vi "Shallow Copy and Deep Copy.vi"() -> ()   [LabVIEW 2020, in "NI_VIAnCFGDataStructure.lvlib" / "Tree.lvclass"]
uses:
  <vilib>/addons/analyzer/VIAnCFGDataStructure/Tree Manager/Tree.lvclass
  <vilib>/addons/analyzer/VIAnCFGDataStructure/Data Types/Int/Int.lvclass/Int.ctl
  <vilib>/addons/analyzer/VIAnCFGDataStructure/Data Types/Path/Path.lvclass/Path.ctl
  <vilib>/addons/analyzer/VIAnCFGDataStructure/Data Types/String/String.lvclass/String.ctl
  <vilib>/addons/analyzer/VIAnCFGDataStructure/Data Types/Path/To Path Tree Data.vi
  <vilib>/addons/analyzer/VIAnCFGDataStructure/Data Types/String/To String Tree Data.vi
  <vilib>/addons/analyzer/VIAnCFGDataStructure/Data Types/Int/To Integer Tree Data.vi
  <vilib>/addons/analyzer/VIAnCFGDataStructure/Data Types/Int/Int.lvclass
  e:/builds/penguin/labview/branches/2020/dev/dist/vi.lib/addons/analyzer/VIAnCFGDataStructure/Tree Data/Tree Data.lvclass
  <vilib>/addons/analyzer/VIAnCFGDataStructure/Data Types/String/String.lvclass
  <vilib>/addons/analyzer/VIAnCFGDataStructure/Data Types/Path/Path.lvclass
  <vilib>/addons/analyzer/VIAnCFGDataStructure/Tree Manager/API/Set Attribute Tree Data.vi
  e:/builds/penguin/labview/branches/2020/dev/dist/vi.lib/addons/analyzer/VIAnCFGDataStructure/Data Types/Int/Int.lvclass
  e:/builds/penguin/labview/branches/2020/dev/dist/vi.lib/addons/analyzer/VIAnCFGDataStructure/Data Types/String/String.lvclass
  e:/builds/penguin/labview/branches/2020/dev/dist/vi.lib/addons/analyzer/VIAnCFGDataStructure/Data Types/Path/Path.lvclass
panel:
  in  "Show IDs (True)":bool
  in  "After Deep Copy":string(tree)
  in  "After Shallow Copy":string(tree)
  in  "Before Copy":string(tree)
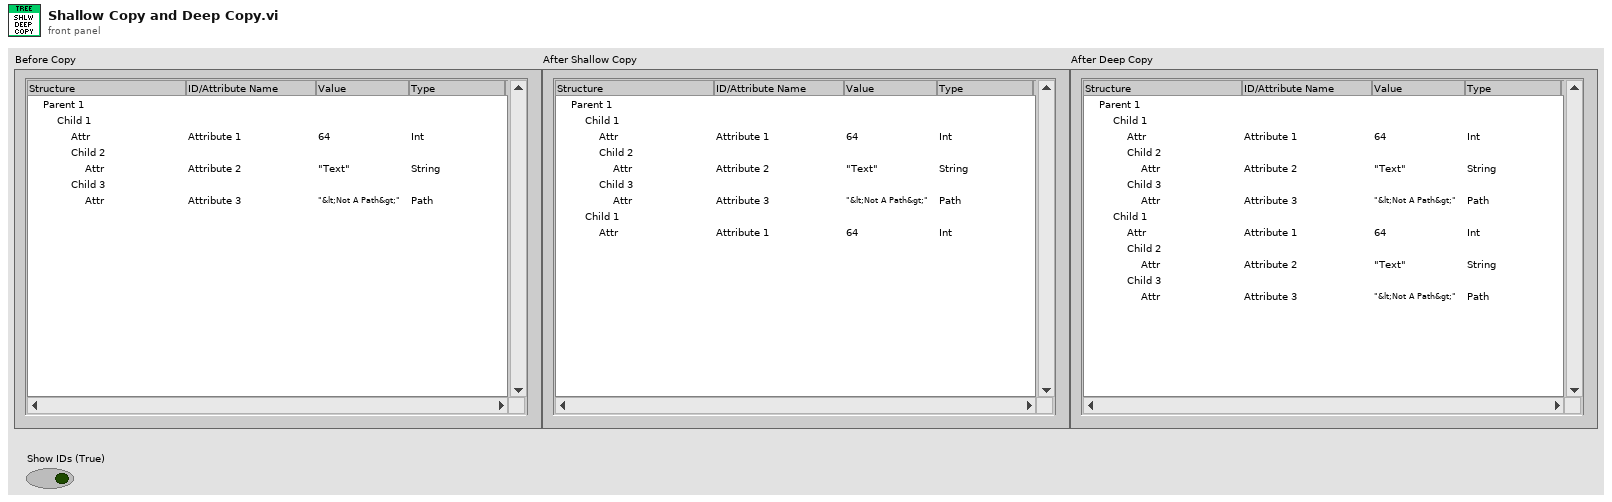
[diagram p1: front panel]
types:
  T1 = typedef "NI_VIAnCFGDataStructure.lvlib/Tree.lvclass/Session Handle.ctl" = refnum<data-value>
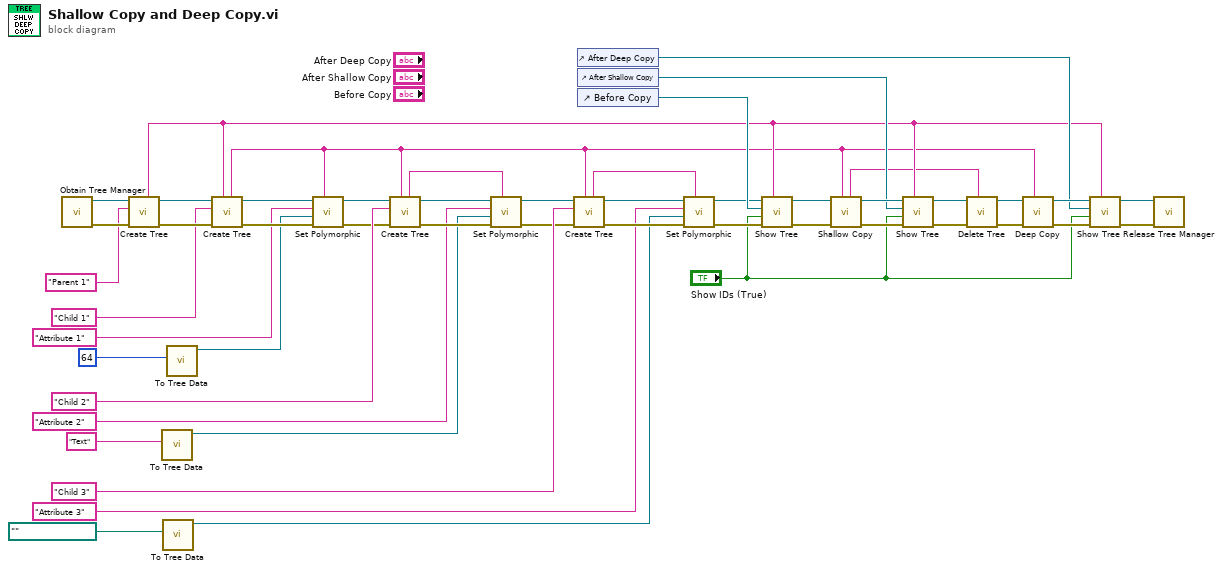
[diagram p0: block diagram]
diagram:
  n1 = call <vilib>:"Obtain Tree Manager.vi"() -> ("Error Out"=w49:errorcluster, "Tree"=w50:T1)  [unwired: 10 in]
  n2 = call <vilib>:"Create Tree.vi"("Error In"=w49, "Name"="Parent 1", "Tree Manager"=w50) -> ("Error Out"=w47:errorcluster, "Tree Manager"=w48:T1, "Unique ID"=w5:string)  [unwired: 6 in]
  n3 = call-poly <vilib>:"To Tree Data.vi"("String"="Text") -> ("String Tree Data"=w12:refnum<class "String.lvclass">)  [unwired: 10 in]
  n4 = call-poly <vilib>:"To Tree Data.vi"("Path"=path "" ("path")) -> ("Path Tree Data"=w10:refnum<class "Path.lvclass">)  [unwired: 10 in]
  n5 = call-poly <vilib>:"To Tree Data.vi"("Integer"=i64 64) -> ("Integer Tree Data"=w15:refnum<class "Int.lvclass">)  [unwired: 10 in]
  n6 = call <vilib>:"Create Tree.vi"("Parent ID (empty)"=w5, "Error In"=w47, "Name"="Child 1", "Tree Manager"=w48) -> ("Error Out"=w21:errorcluster, "Tree Manager"=w23:T1, "Unique ID"=w4:string)  [unwired: 5 in]
  n7 = call-poly <vilib>:"Set Polymorphic.vi"("Tree ID"=w4, "Error In"=w21, "Attribute Value"=w15, "Attribute Name"="Attribute 1", "Tree Manager"=w23) -> ("Error Out"=w20:errorcluster, "Tree Manager"=w22:T1)  [unwired: 4 in, 1 out]
  n8 = call <vilib>:"Create Tree.vi"("Parent ID (empty)"=w4, "Error In"=w20, "Name"="Child 2", "Tree Manager"=w22) -> ("Error Out"=w24:errorcluster, "Tree Manager"=w27:T1, "Unique ID"=w3:string)  [unwired: 5 in]
  n9 = call-poly <vilib>:"Set Polymorphic.vi"("Tree ID"=w3, "Error In"=w24, "Attribute Value"=w12, "Attribute Name"="Attribute 2", "Tree Manager"=w27) -> ("Error Out"=w25:errorcluster, "Tree Manager"=w26:T1)  [unwired: 4 in, 1 out]
  n10 = call <vilib>:"Create Tree.vi"("Parent ID (empty)"=w4, "Error In"=w25, "Name"="Child 3", "Tree Manager"=w26) -> ("Error Out"=w28:errorcluster, "Tree Manager"=w29:T1, "Unique ID"=w2:string)  [unwired: 5 in]
  n11 = control-ref of="After Deep Copy"() -> (w7:refnum<vi>)
  n12 = control-ref of="After Shallow Copy"() -> (w8:refnum<vi>)
  n13 = control-ref of="Before Copy"() -> (w44:refnum<vi>)
  n14 = call-poly <vilib>:"Set Polymorphic.vi"("Tree ID"=w2, "Error In"=w28, "Attribute Value"=w10, "Attribute Name"="Attribute 3", "Tree Manager"=w29) -> ("Error Out"=w18:errorcluster, "Tree Manager"=w19:T1)  [unwired: 4 in, 1 out]
  n15 = call <vilib>:"Show Tree.vi"("Root ID"=w5, "Error In"=w18, "Show IDs (False)"="Show IDs (True)", "Tree Ref"=w44, "Tree"=w19) -> ("Error Out"=w40:errorcluster, "Tree"=w41:T1)  [unwired: 5 in]
  n16 = call <vilib>:"Shallow Copy.vi"("Tree ID"=w4, "Error In"=w40, "Tree Manager"=w41) -> ("Error Out"=w38:errorcluster, "Tree Manager"=w39:T1, "Unique ID of Copied Tree"=w1:string)  [unwired: 6 in]
  n17 = call <vilib>:"Show Tree.vi"("Root ID"=w5, "Error In"=w38, "Show IDs (False)"="Show IDs (True)", "Tree Ref"=w8, "Tree"=w39) -> ("Error Out"=w36:errorcluster, "Tree"=w37:T1)  [unwired: 5 in]
  n18 = call <vilib>:"Delete Tree.vi"("Tree ID"=w1, "Error In"=w36, "Tree Manager"=w37) -> ("Error Out"=w34:errorcluster, "Tree Manager"=w35:T1)  [unwired: 7 in]
  n19 = call <vilib>:"Deep Copy.vi"("Tree ID"=w4, "Error In"=w34, "Tree Manager"=w35) -> ("Error Out"=w32:errorcluster, "Tree Manager"=w33:T1)  [unwired: 6 in, 1 out]
  n20 = call <vilib>:"Show Tree.vi"("Root ID"=w5, "Error In"=w32, "Show IDs (False)"="Show IDs (True)", "Tree Ref"=w7, "Tree"=w33) -> ("Error Out"=w30:errorcluster, "Tree"=w31:T1)  [unwired: 5 in]
  n21 = call <vilib>:"Release Tree Manager.vi"("Error In"=w30, "Tree"=w31) -> ()  [unwired: 9 in, 1 out]
